vi "Read controlInfo.vi"(8 "error in (no error)":errorcluster, 11 "Enumeration in":refnum<class "Enumeration.lvclass">) -> (0 "error out":errorcluster, 2 "ControlInfo":T1, 3 "Enumeration out":refnum<class "Enumeration.lvclass">)   [LabVIEW 2016, in "Enumeration.lvclass"]
uses:
  Enumeration.lvclass
  Typedefs/ControlInfo.ctl
  Enumeration.lvclass/Enumeration.ctl
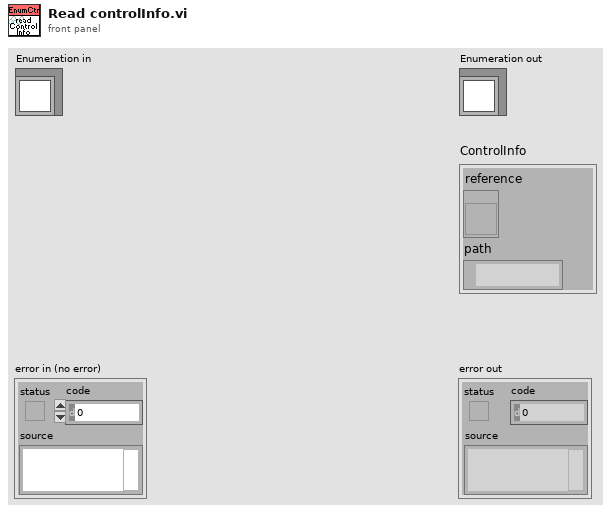
[diagram p1: front panel]
types:
  T1 = typedef "ControlInfo.ctl" = cluster{"reference":refnum<vi>, "path":path}
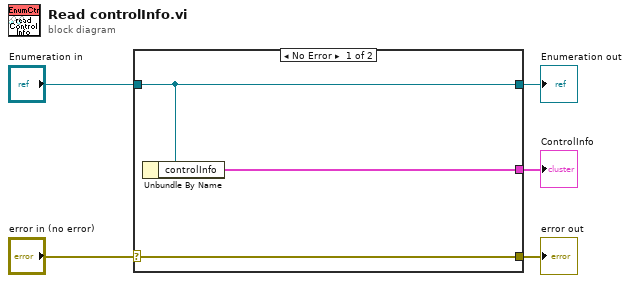
[diagram p0: block diagram]
diagram:
  n1 = case shown="No Error" "error in (no error)" {
    selector: "error in (no error)" -> [w8 w9]
    tunnel: [w8 w9] -> w4
    tunnel: [w7 w10] -> w2
    tunnel: "Enumeration in" -> [w7 w10]
    tunnel: [w6 _] -> w1
    frame No Error {
      n2 = Unbundle By Name(w7) -> ("controlInfo"=w6:T1)
    }
    frame Error {
    }
  }
  "error out" <- w4
  "Enumeration out" <- w2
  "ControlInfo" <- w1
